vi "Publish.vi"(0 "String":string, 2 "Topic":string="/junk", 3 "node":string) -> (1 "error":errorcluster)   [LabVIEW 2012]
doc: "Starts a publisher on the RIO"
uses:
  <userlib>/ROSforLV/ROS/Code/Console/Servers/ServerSubs/TopicDef.ctl
  <userlib>/ROSforLV/ROS/Code/SubVIs/_ROSDirection.ctl
  <userlib>/ROSforLV/ROS/MessageBuilding/std_msgs/subs/stringScalar.vi
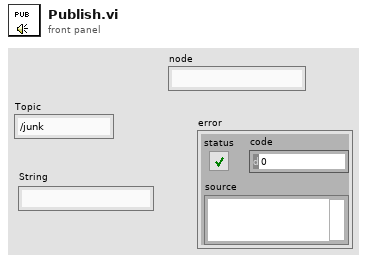
[diagram p1: front panel]
types:
  T1 = typedef "TopicDef.ctl" = cluster{"Topic":string, "Type":string, "Action":T2, "Update (ms)":u16, "queue size":u16}
  T2 = typedef "_ROSDirection.ctl" = enum16{"Node", "Publisher", "Subscriber", "Service Client"}
  T3 = typedef "_ROSControl.ctl" = cluster{"topic port":u16, "Node":string, "topic":string, "type":string, "node port":u16, "error ":errorcluster, "Direction":T2, "Update (ms)":u16, "queue size":u16}
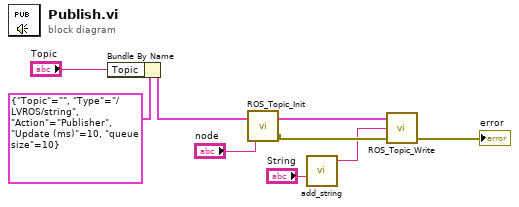
[diagram p0: block diagram]
diagram:
  n1 = Bundle By Name(cluster=T1 {"Topic"="", "Type"="/LVROS/string", "Action"=enum."Publisher", "Update (ms)"=10, "queue size"=10} ("Definitions"), "Topic"="Topic") -> (w5:T1)
  n2 = call <userlib>:"ROS_Topic_Init.vi"("node"="node", "Definitions"=w5) -> ("error out"=w2:errorcluster, "ROS out"=w9:T3)
  n3 = call-poly <userlib>:"add_string.vi"("String"="String") -> ("msg out"=w1:string)  [unwired: 4 in]
  n4 = call <userlib>:"ROS_Topic_Write.vi"("error in (no error)"=w2, "Msg in"=w1, "ROS in"=w9) -> ("error out"=→"error":errorcluster)  [unwired: 1 in, 1 out]
